vi "On Stop Motion (SubVI).vi"(0 "CmdLib In":refnum<k24>, 5 "Device Address In":i32, 7 "Motor":i32, 9 "DeviceKey In":string, 11 "error in":errorcluster) -> (4 "CmdLib In Out":refnum<k24>, 15 "error out":errorcluster)   [LabVIEW 2017]
doc: "by Tanguy BOULARD"
uses:
  dll/CmdLib.dll
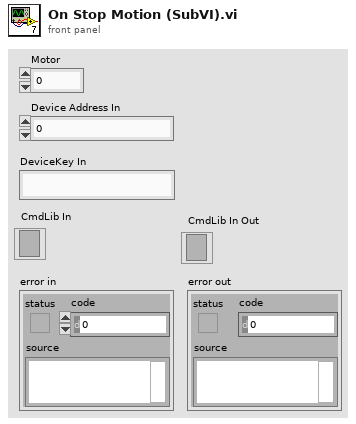
[diagram p1: front panel]
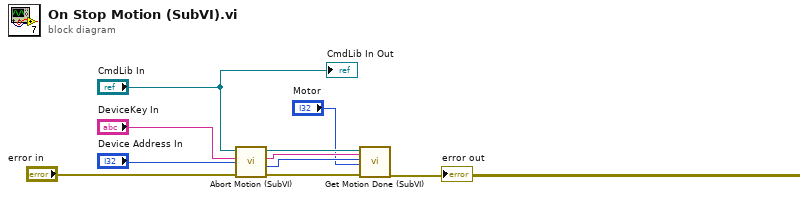
[diagram p0: block diagram]
diagram:
  n1 = call "Abort Motion (SubVI).vi"("error in (no error)"="error in", "Device Address In"="Device Address In", "DeviceKey In"="DeviceKey In", "CmdLib In"="CmdLib In") -> ("error out"=w8:errorcluster, "Device Address Out"=w7:i32, "DeviceKey Out"=w6:string, "CmdLib Out"=w5:refnum<k24>)
  n2 = call "Get Motion Done (SubVI).vi"("CmdLib In"=w5, "DeviceKey In"=w6, "Device Address In"=w7, "Motor"="Motor", "error in (no error)"=w8) -> ("error out"=→"error out":errorcluster)  [unwired: 10 in, 4 out]
  "CmdLib In Out" <- "CmdLib In"
